vi "Leg Controller.vi"(8 "error in":errorcluster) -> ()   [LabVIEW 2018]
doc: "This VI executes continuously carrying out the current operation and responding to updates or new operations. It will often contain the timing or control code that is difficult to place directly in TeleOp. This VI generally opens all sensors and motors and isolates the rest of the robot code from knowing how the operations are carried out."
uses:
  <vilib>/Rock Robotics/WPI/Framework/Completion Status.ctl
  Leg Setpoints.ctl
  Leg Operations.ctl
  <vilib>/Rock Robotics/WPI/Solenoid/WPI_SolenoidValue.ctl
  <vilib>/Rock Robotics/WPI/Solenoid/WPI_SolenoidDevRef.ctl
  <vilib>/Rock Robotics/WPI/Solenoid/WPI_SolenoidChannel.ctl
  <vilib>/Rock Robotics/WPI/Solenoid/WPI_SolenoidSetEnum.vi
  <vilib>/Rock Robotics/Network Tables/NT Write Boolean.vi
panel:
  in  "PositionValue":T1=enum."Reverse"
  in  "Interactive Values":T2
  out "Current\nCmd":string="Started at  08:52:34.924\n: Reserve,  S 0.0, D 0.000000"
  in  "Buttons":cluster{"Execute Cmd":bool, "Abort Cmd":bool}
  out "Command Timing":cluster{"Start Time (ms)":u32, "Iterations":i32}={"Start Time (ms)"=697524, "Iterations"=0}
  out "Status":T4
  # "Tip: It may be helpful to observe inputs and sensor values.\nYou may also want to display tuning or debugging controls."
  # "Interactive Command: You may fill in the settings for a command\nand schedule it with the Execute button. You can observe and abort\nany command while fine tuning the code for the controller."
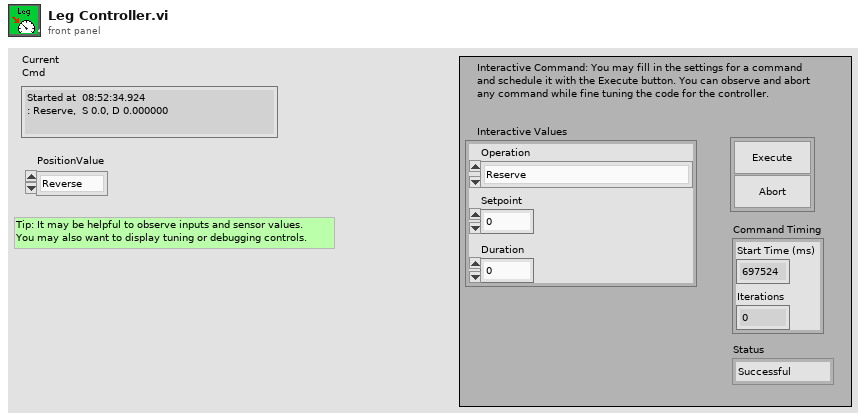
[diagram p1: front panel]
types:
  T1 = typedef "WPI_SolenoidValue.ctl" = enum16{"Off", "On", "Forward", "Reverse"}
  T2 = typedef "Leg Setpoints.ctl" = cluster{"Operation":T3, "Setpoint":dbl, "Duration":dbl}
  T3 = typedef "Leg Operations.ctl" = enum16{"Reserve", "Read Current", "Immediate", "Release"}
  T4 = typedef "Completion Status.ctl" = enum16{"Successful", "Aborted", "Incomplete"}
  T5 = typedef "WPI_SolenoidDevRef.ctl" = cluster{"DevStatus":errorcluster, "Pneumatics Control Module":u8, "Forward Solenoid Channel":T6, "Reverse Solenoid Channel":T6}
  T6 = typedef "WPI_SolenoidChannel.ctl" = enum8{"Solenoid 0", "Solenoid 1", "Solenoid 2", "Solenoid 3", "Solenoid 4", "Solenoid 5", "Solenoid 6", "Solenoid 7", "Invalid"}
  T7 = typedef "Command Status Info.ctl" = cluster{"Name":string, "Status":T4, "notifier out":T8}
  T8 = typedef "Completion Notifier.ctl" = refnum<notifier>
  T9 = cluster{"Current Command":T2, "Command Timing":cluster{"Start Time (ms)":u32, "Iterations":i32}, "Command Arguments":cluster{"Command Info":T7, "Description":string, "Default Command":T2, "queue out":refnum<queue>, "Subsystem Name":string}}
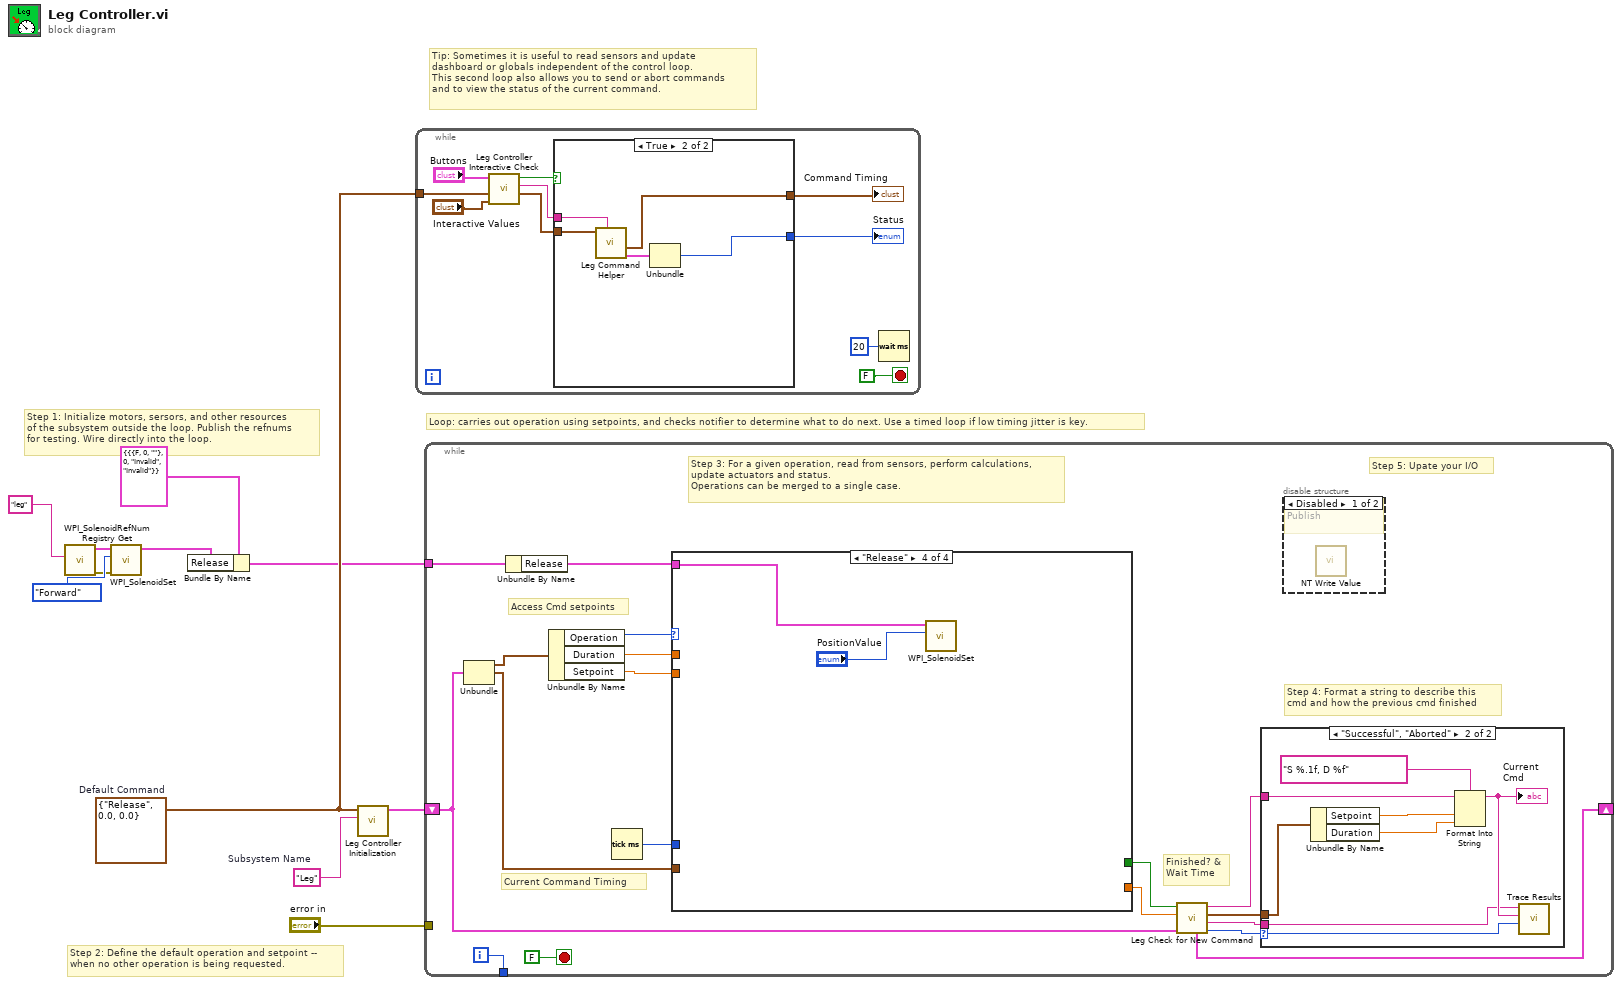
[diagram p0: block diagram]
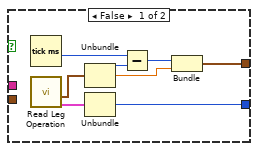
[diagram p2: hidden frame]
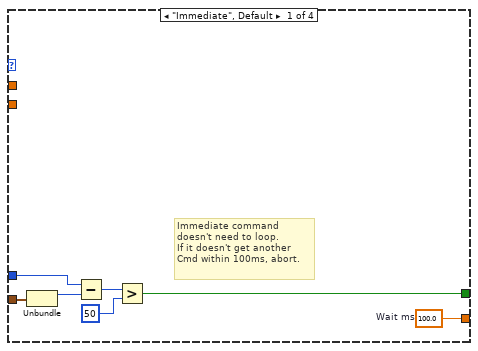
[diagram p5: hidden frame]
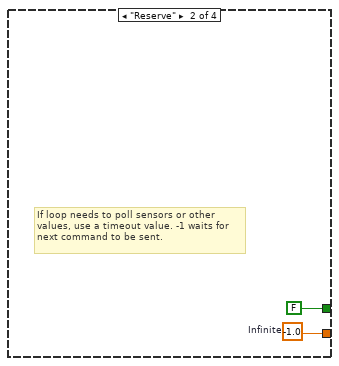
[diagram p6: hidden frame]
diagram:
  w8 = T2 {"Operation"=enum."Release", "Setpoint"=0.0, "Duration"=0.0}  # Default Command
  w9 = "Leg"  # Subsystem Name
  # "Tip: Sometimes it is useful to read sensors and update\ndashboard or globals independent of the control loop.\nThis second loop also allows you to send or abort commands\nand to view the status of the current command."
  # "Step 2: Define the default operation and setpoint --\nwhen no other operation is being requested."
  # "Step 1: Initialize motors, sersors, and other resources\nof the subsystem outside the loop. Publish the refnums\nfor testing. Wire directly into the loop."
  # "Loop: carries out operation using setpoints, and checks notifier to determine what to do next. Use a timed loop if low timing jitter is key."
  n1 = call <vilib>:"WPI_SolenoidRefNum Registry Get.vi"("refnum name"="leg") -> ("error out"=w3:errorcluster, "SolenoidDevRef"=w2:T5)  [unwired: 9 in]
  n2 = call-poly <vilib>:"WPI_SolenoidSet.vi"("error in (no error)"=w3, "Value"=WPI_SolenoidValue."Forward", "SolenoidDevRef"=w2) -> ("SolenoidDevRef"=w7:T5)  [unwired: 7 in, 1 out]
  n3 = Bundle By Name(cluster=cluster{"Release":T5} {"Release"={"DevStatus"={"status"=FALSE, "code"=0, "source"=""}, "Pneumatics Control Module"=0, "Forward Solenoid Channel"=enum."Invalid", "Reverse Solenoid Channel"=enum."Invalid"}} ("input cluster"), "Release"=w7) -> (w4:cluster{"Release":T5})
  n4 = call "Leg Controller Initialization.vi"("Subsystem Name"=w9, "Default Command"=w8) -> ("Current Command"=w10:T9)  [unwired: 9 in]
  n5 = while {
    tunnel: w8 -> [w18]
    stop <- FALSE stop-if-true
    n6 = call "Leg Controller Interactive Check.vi"("Interactive Command in"="Interactive Values", "Default Command"=w18, "Buttons"="Buttons") -> ("Interactive Command out"=w15:T2, "Trace String"=w16:string, "Schedule"=w17:bool)  [unwired: 6 in]
    n7 = case shown="True" w17 {
      tunnel: [w29 w34] -> w14
      tunnel: w15 -> [_ w32]
      tunnel: [w25 w30] -> w13
      tunnel: w16 -> [_ w33]
      frame False {
        n8 = Tick Count (ms)() -> (millisecond timer value=w24:u32)
        n9 = call "Read Leg Operation.vi"() -> ("Command Info"=w22:T7, "SubSystem Data"=w23:T2)  [unwired: 9 in, 1 out]
        n10 = Unbundle(w23) -> ("Operation"=w28:T3, "Setpoint"=w26:dbl)  [unwired: 1 out]
        n11 = Unbundle(w22) -> ("Status"=w29:T4)  [unwired: 2 out]
        n12 = Subtract(x=w24, y=w28) -> (x-y=w27:u32)
        n13 = Bundle(w27, "Setpoint"=w26) -> (w25:cluster{u32, "Setpoint":dbl})  [unwired: 1 in]
      }
      frame True {
        n14 = call "Leg Command Helper.vi"("Description"=w33, "SubSystem Data"=w32) -> ("Command Info Out"=w31:T7, "Command Timing"=w30:cluster{"Start Time (ms)":u32, "Iterations":i32})  [unwired: 7 in, 1 out]
        n15 = Unbundle(w31) -> ("Status"=w34:T4)  [unwired: 2 out]
      }
    }
    "Status" <- w14
    "Command Timing" <- w13
    n16 = Wait (ms)(milliseconds to wait=u32 20) -> ()  [unwired: 1 out]
  }
  n17 = while {
    shift-right: [w44] -> _
    shift-left: w10 -> [w37]
    tunnel: [w51] -> _
    tunnel: "error in" -> [_]
    tunnel: w4 -> [w36]
    i -> [w51]
    stop <- FALSE stop-if-true
    # "Step 5: Upate your I/O"
    # "Step 4: Format a string to describe this\ncmd and how the previous cmd finished"
    # "Current Command Timing"
    # "Access Cmd setpoints"
    # "Finished? &\nWait Time"
    # "Step 3: For a given operation, read from sensors, perform calculations,\nupdate actuators and status.\nOperations can be merged to a single case."
    n18 = Unbundle(w37) -> ("Current Command"=w50:T2, "Command Timing"=w46:cluster{"Start Time (ms)":u32, "Iterations":i32})  [unwired: 1 out]
    n19 = Unbundle By Name(w36) -> ("Release"=w35:T5)
    n20 = Unbundle By Name(w50) -> ("Operation"=w49:T3, "Duration"=w48:dbl, "Setpoint"=w45:dbl)
    n21 = Tick Count (ms)() -> (millisecond timer value=w47:u32)
    n22 = case shown="\"Release\"" w49 {
      tunnel: [w67 w69 _ _] -> w42
      tunnel: [w61 FALSE ("ignore previous (F)") _ _] -> w43
      tunnel: w46 -> [w63 _ _ _]
      tunnel: w48 -> [_ _ _ _]
      tunnel: w47 -> [w62 _ _ _]
      tunnel: w45 -> [_ _ _ _]
      tunnel: w35 -> [_ _ _ w71]
      frame "Immediate", Default {
        w67 = 100.0  # Wait ms
        # "Immediate command\ndoesn't need to loop.\nIf it doesn't get another\nCmd within 100ms, abort."
        n23 = Unbundle(w63) -> ("Start Time (ms)"=w66:u32)  [unwired: 1 out]
        n24 = Subtract(x=w62, y=w66) -> (x-y=w65:u32)
        n25 = Greater?(x=w65, y=u8 50 ("Left Motor")) -> (0:w61:bool)
      }
      frame "Reserve" {
        w69 = -1.0  # Infinite
        # "If loop needs to poll sensors or other\nvalues, use a timeout value. -1 waits for\nnext command to be sent."
      }
      frame "Read Current" {
      }
      frame "Release" {
        n26 = call-poly <vilib>:"WPI_SolenoidSet.vi"("Value"="PositionValue", "SolenoidDevRef"=w71) -> ()  [unwired: 8 in, 2 out]
      }
    }
    n27 = call "Leg Check for New Command.vi"("Current Command"=w37, "Wait time (ms)"=w42, "Finished?"=w43) -> ("Completion"=w38:T4, "Subsystem Name"=w39:string, "Current Command"=w40:T2, "Initial Trace String"=w41:string, "NextCommand"=w44:T9)  [unwired: 4 in]
    n28 = case shown="\"Successful\", \"Aborted\"" w38 {
      selector: w38 -> [_ w60]
      tunnel: w41 -> [_ w56]
      tunnel: w40 -> [_ w57]
      tunnel: w39 -> [_ w53]
      frame "Incomplete", Default {
        # "Continuing current command"
      }
      frame "Successful", "Aborted" {
        # "Report and setup for next command"
        n29 = Unbundle By Name(w57) -> ("Setpoint"=w59:dbl, "Duration"=w54:dbl)
        n30 = Format Into String(format string="S %.1f, D %f", initial string=w56, w59, w54) -> (resulting string=w55:string)  [unwired: 1 in, 1 out]
        "Current\nCmd" <- w55
        n31 = call <vilib>:"Trace Results.vi"("Status of previous command"=w60, "Description"=w55, "Subsystem"=w53) -> ()  [unwired: 9 in]
      }
    }
    n32 = disable-structure shown="Disabled" {
      frame Disabled {
        # "Publish"
        n33 = call-poly <vilib>:"NT Write Value.vi"() -> ()  [unwired: 11 in, 1 out]
      }
      frame Enabled {
      }
    }
  }
